vi "LV2 Global Performance Test.vi"() -> ()   [LabVIEW 2021]
panel:
  out "x-y":dbl format="%#_6p"
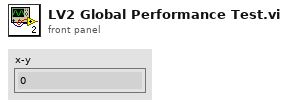
[diagram p1: front panel]
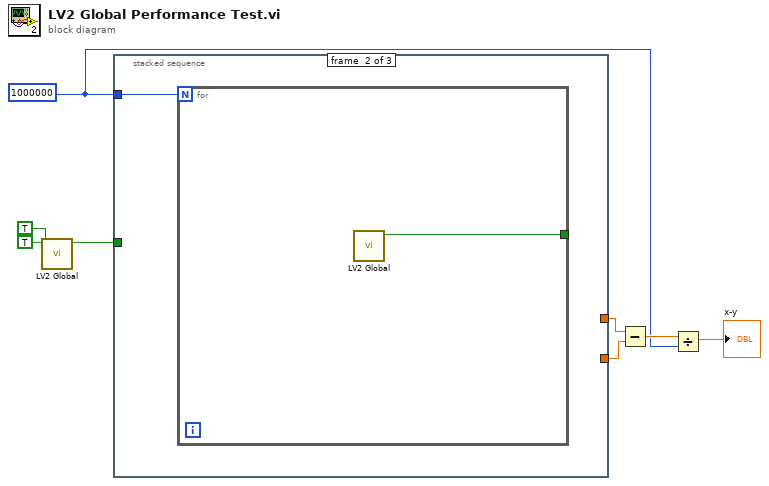
[diagram p0: block diagram]
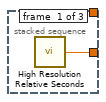
[diagram p2: hidden frame]
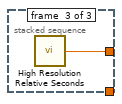
[diagram p3: hidden frame]
diagram:
  w4 = 1000000
  n1 = call "LV2 Global.vi"("Write"=TRUE, "Boolean In"=TRUE) -> ("Boolean"=w2:bool)  [unwired: 9 in]
  n2 = stacked-sequence {
    tunnel: [w9 _ _] -> w8
    tunnel: [_ _ w12] -> w7
    tunnel: w4 -> [_ w10 _]
    tunnel: w2 -> [_ _ _]
    frame #0 {
      n3 = call <vilib>:"High Resolution Relative Seconds.vi"() -> ("relative seconds"=w9:dbl)
    }
    frame #1 {
      n4 = for {
        N: w10 -> [_]
        tunnel: [w11] -> _
        n5 = call "LV2 Global.vi"() -> ("Boolean"=w11:bool)  [unwired: 11 in]
      }
    }
    frame #2 {
      n6 = call <vilib>:"High Resolution Relative Seconds.vi"() -> ("relative seconds"=w12:dbl)
    }
  }
  n7 = Subtract(x=w7, y=w8) -> (x-y=w6:dbl)
  n8 = Divide(x=w6, y=w4) -> (x/y=→"x-y":dbl)
